vi "24-2.vi"() -> ()   [LabVIEW 2019, in "24.lvlib"]
uses:
  24.lvlib
panel:
  out "Min Model No.":u64
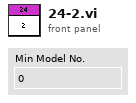
[diagram p1: front panel]
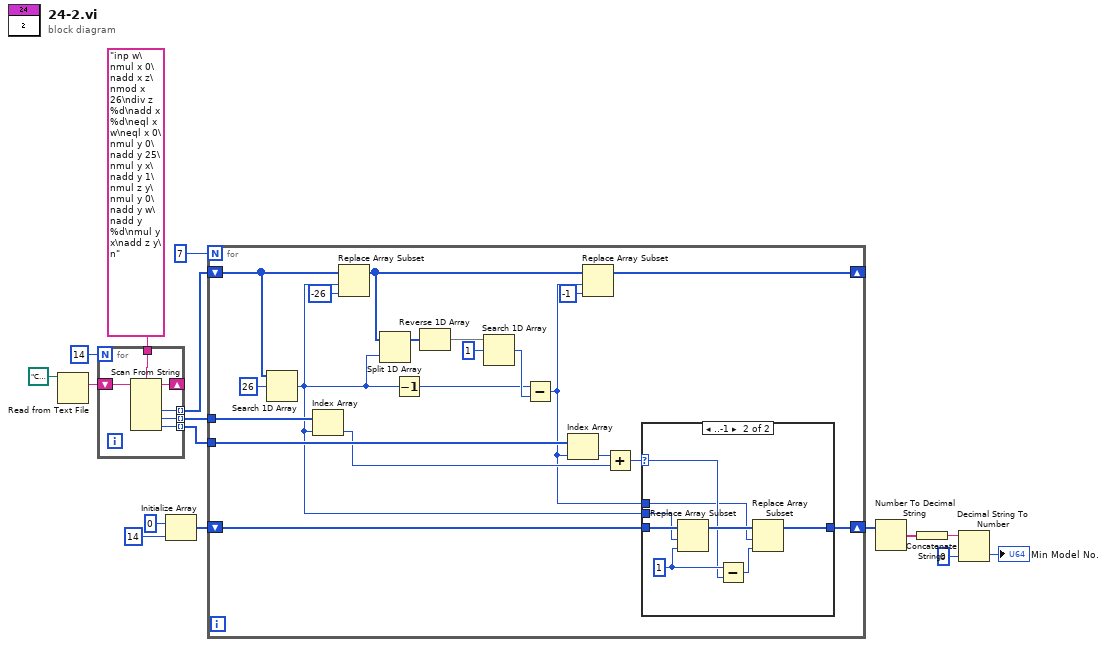
[diagram p0: block diagram]
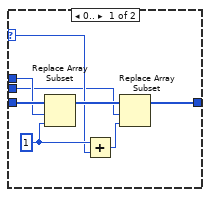
[diagram p2: hidden frame]
diagram:
  n1 = Read from Text File(file (use dialog)=path "C:/Users/craig.walker/Documents/GitHub/lv2019-Advent-of-Code-2021/24/input.txt") -> (text=w16:string)  [unwired: 3 in, 3 out]
  n2 = for {
    N: 14 -> [_]
    tunnel: "inp w\nmul x 0\nadd x z\nmod x 26\ndiv z %d\nadd x %d\neql x w\neql x 0\nmul y 0\nadd y 25\nmul y x\nadd y 1\nmul z y\nmul y 0\nadd y w\nadd y %d\nmul y x\nadd z y\n" ("format string") -> [w21]
    tunnel: [w20] -> w11 mode=indexing
    tunnel: [w19] -> w10 mode=indexing
    tunnel: [w18] -> w9 mode=indexing
    shift-right: [w17] -> _
    shift-left: w16 -> [w22]
    n3 = Scan From String(format string=w21, input string=w22) -> (remaining string=w17:string, output 1=w20:i32, output 2=w19:i32, output 3=w18:i32)  [unwired: 5 in, 2 out]
  }
  n4 = Initialize Array(0 ("element"), 14 ("dimension size")) -> (w6:i32[])
  n5 = for {
    N: 7 -> [_]
    shift-right: [w32] -> _
    shift-left: w11 -> [w40]
    shift-right: [w23] -> w5
    shift-left: w6 -> [w41]
    tunnel: w10 -> [w30]
    tunnel: w9 -> [w29]
    n6 = Search 1D Array(1D array=w40, element=26) -> (index of element=w26:i32)  [unwired: 1 in]
    n7 = Index Array(array=w30, index=w26) -> (element=w27:i32)
    n8 = Replace Array Subset(array=w40, new element=-26 ("new element/subarray"), index=w26) -> (w33:i32[])
    n9 = Split 1D Array(array=w33, index=w26) -> (first subarray=w38:i32[])  [unwired: 1 out]
    n10 = Decrement(x=w26) -> (x-1=w34:i32)
    n11 = Reverse 1D Array(array=w38) -> (reversed array=w37:i32[])
    n12 = Search 1D Array(1D array=w37, element=1) -> (index of element=w35:i32)  [unwired: 1 in]
    n13 = Subtract(x=w34, y=w35) -> (x-y=w25:i32)
    n14 = Index Array(array=w29, index=w25) -> (element=w28:i32)
    n15 = Replace Array Subset(array=w33, new element=-1 ("new element/subarray"), index=w25) -> (w32:i32[])
    n16 = Add(x=w28, y=w27) -> (x+y=w24:i32)
    n17 = case shown="..-1" w24 {
      selector: w24 -> [w47 w55]
      tunnel: w41 -> [w50 w58]
      tunnel: w26 -> [w43 w52]
      tunnel: w25 -> [w44 w51]
      tunnel: [w45 w53] -> w23
      frame 0.. {
        w48 = 1 ("new element/subarray")
        n18 = Replace Array Subset(array=w50, new element=w48, index=w44) -> (w49:i32[])
        n19 = Add(x=w48, y=w47) -> (x+y=w46:i32)
        n20 = Replace Array Subset(array=w49, new element=w46, index=w43) -> (w45:i32[])
      }
      frame ..-1 {
        w56 = 1 ("new element/subarray")
        n21 = Replace Array Subset(array=w58, new element=w56, index=w52) -> (w57:i32[])
        n22 = Subtract(x=w56, y=w55) -> (x-y=w54:i32)
        n23 = Replace Array Subset(array=w57, new element=w54, index=w51) -> (w53:i32[])
      }
    }
  }
  n24 = Number To Decimal String(number=w5) -> (decimal integer string=w4:string[])  [unwired: 1 in]
  n25 = Concatenate Strings(w4) -> (w3:string)
  n26 = Decimal String To Number(string=w3, default (0L)=u64 0 ("default (0 I32)")) -> (number=→"Min Model No.":u64)  [unwired: 1 in, 1 out]
